vi "LabVIEW 2.vi"() -> ()   [LabVIEW 2020]
panel:
  in  "Commande stop structure":bool
  out "Indicateur evenement":bool
  out "Affichage condition 2":string
  in  "Commande condition num":i32
  out "Iterateur for":i32
  in  "Nombre d'itération boucle for":i32
  out "Iterateur while":i32
  in  "Commande while":bool
  out "Affichage condition 1":string
  in  "Commande structure if":bool
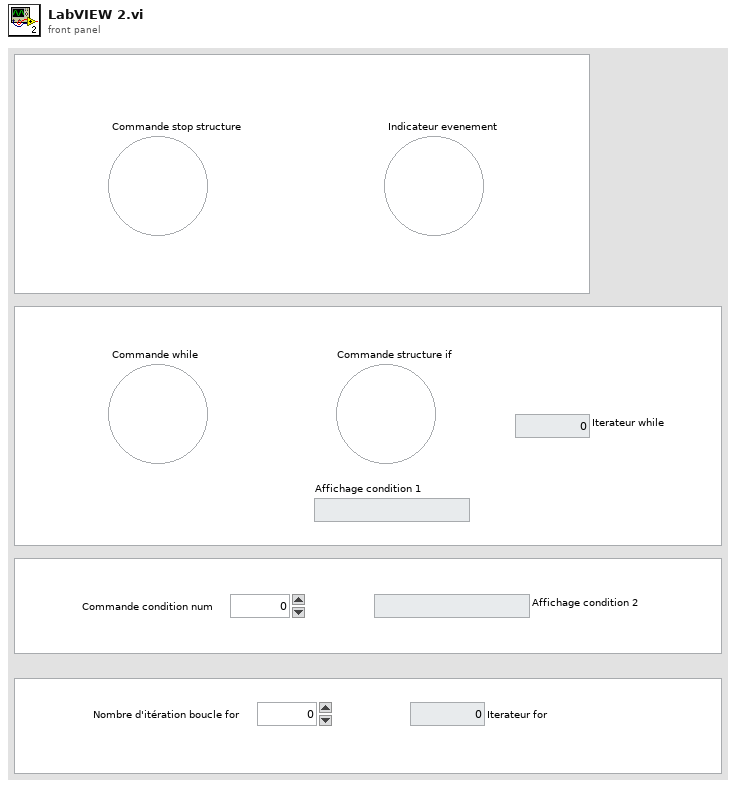
[diagram p1: front panel]
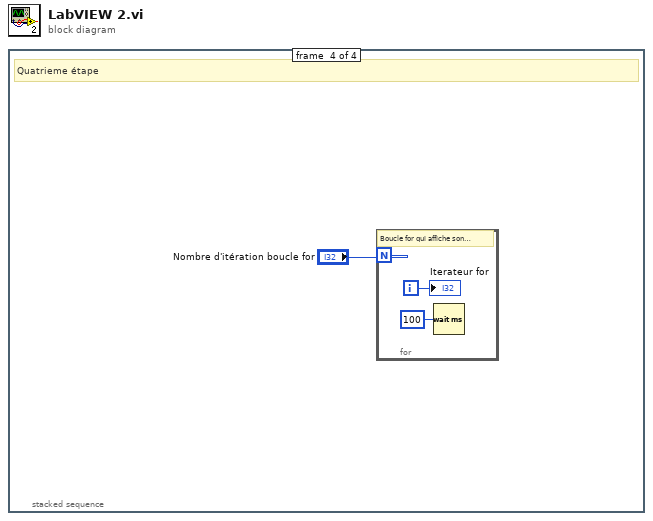
[diagram p0: block diagram]
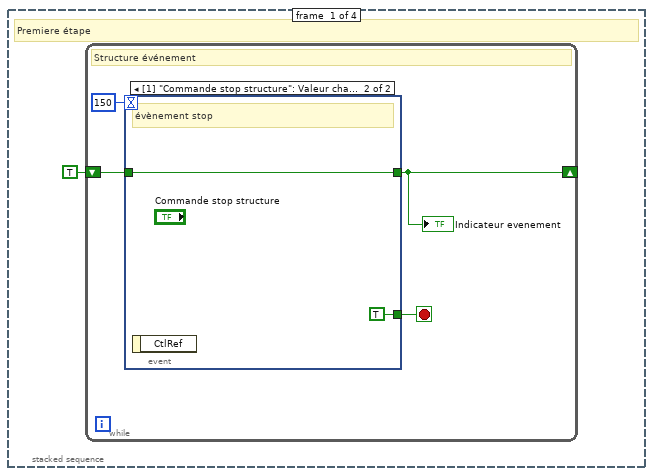
[diagram p2: hidden frame]
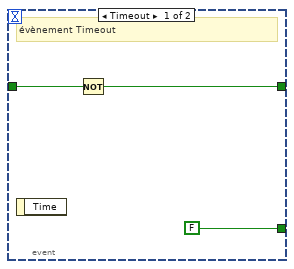
[diagram p3: hidden frame]
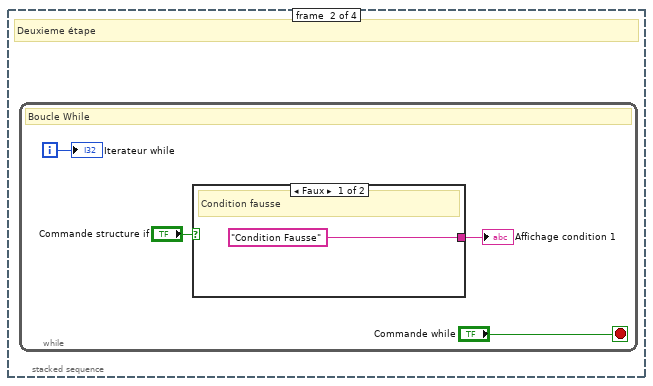
[diagram p4: hidden frame]
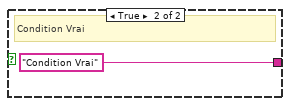
[diagram p5: hidden frame]
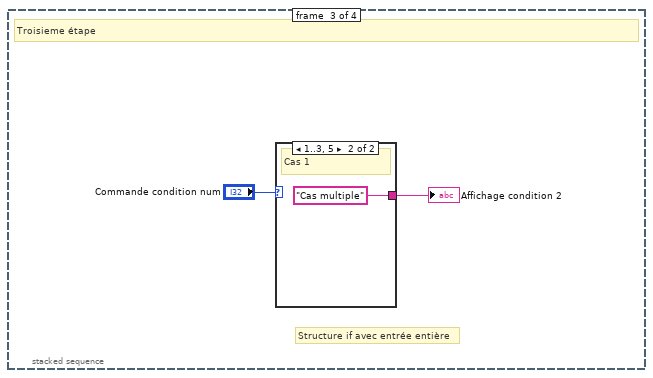
[diagram p6: hidden frame]
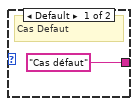
[diagram p7: hidden frame]
diagram:
  n1 = stacked-sequence {
    frame #0 {
      # "Premiere étape"
      n2 = while {
        shift-right: [w3] -> _
        shift-left: TRUE -> [w4]
        stop <- w2 stop-if-true
        # "Structure événement"
        n3 = event shown="[1] \"Commande stop structure\": Valeur changée" {
          selector: _ -> [_ _]
          dyn-events: _ -> [_ _]
          timeout: 150 -> [_ _]
          tunnel: w4 -> [w8 w10]
          tunnel: [w7 w10] -> w3
          tunnel: [FALSE TRUE] -> w2
          event Timeout {
            # "évènement Timeout"
            n4 = event-data() -> ()  [unwired: 1 in, 1 out]
            n5 = Not(x=w8) -> (.not. x?=w7:bool)
          }
          event "Commande stop structure": Value Change {
            # "évènement stop"
            n6 = event-data() -> ()  [unwired: 1 in, 1 out]
          }
        }
        "Indicateur evenement" <- w3
      }
    }
    frame #1 {
      # "Deuxieme étape"
      n7 = while {
        i -> [w11]
        stop <- "Commande while" stop-if-true
        # "Boucle While"
        n8 = case shown="Faux" "Commande structure if" {
          tunnel: ["Condition Fausse" "Condition Vrai"] -> w13
          frame False {
            # "Condition fausse"
          }
          frame True {
            # "Condition Vrai"
          }
        }
        "Affichage condition 1" <- w13
        "Iterateur while" <- w11
      }
    }
    frame #2 {
      # "Structure if avec entrée entière"
      # "Troisieme étape"
      n9 = case shown="1..3, 5" "Commande condition num" {
        tunnel: ["Cas défaut" "Cas multiple"] -> w18
        frame Default {
          # "Cas Defaut"
        }
        frame 1..3, 5 {
          # "Cas 1"
        }
      }
      "Affichage condition 2" <- w18
    }
    frame #3 {
      # "Quatrieme étape"
      n10 = for {
        N: "Nombre d'itération boucle for" -> [_]
        i -> [w23]
        # "Boucle for qui affiche son itérateur"
        n11 = Wait (ms)(milliseconds to wait=u32 100 ("attente (ms)")) -> ()  [unwired: 1 out]
        "Iterateur for" <- w23
      }
    }
  }
